vi "DSF.Engine.Transfer.Create.vi"(5 "id":i32, 7 "channel blocks":T1[](array[typedef]) {"buffer offset" format="%d bytes"}, 8 "error in (no error)":errorcluster, 9 "String Buffer":refnum<class "DSF.Engine.Memory.Buffer.lvclass">, 10 "Intermediate Buffer":refnum<class "DSF.Engine.Pointer.DBL.lvclass">, 11 "Inline Buffer":refnum<class "DSF.Engine.Pointer.DBL.lvclass">) -> (0 "error out":errorcluster, 3 "Transfer out":refnum<class "DSF.Engine.Transfer.lvclass">)   [LabVIEW 2017, in "DSF.Engine.lvlib" / "DSF.Engine.Transfer.lvclass"]
uses:
  DSF.Engine.Transfer.lvclass
  Buffer/DSF.Engine.Memory.Buffer.lvclass
  Pointer/DSF.Engine.Pointer.DBL.lvclass
  Shared/Typedefs/DSF Runtime Channel Block.ctl
  DSF Configuration API/1.0.0/Public/Controls/DSF Data Type.ctl
  DSF.Engine.Transfer.lvclass/DSF.Engine.Transfer.ctl
  DSF.Engine.lvlib
  DSF Configuration API/1.0.0/DSF Configuration API.lvlib
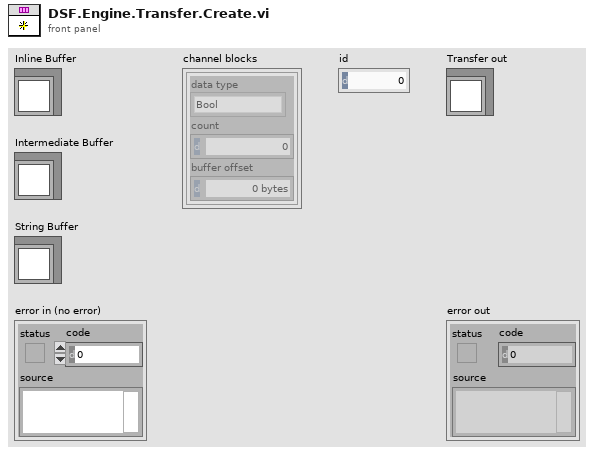
[diagram p1: front panel]
types:
  T1 = typedef "DSF.Engine.lvlib/DSF Runtime Channel Block.ctl" = cluster{"data type":T2, "count":u64, "buffer offset":u64}
  T2 = typedef "DSF Configuration API.lvlib/DSF Data Type.ctl" = enum8{"Bool", "SGL", "DBL", "I8", "I16", "I32", "I64", "U8", "U16", "U32", "U64"}
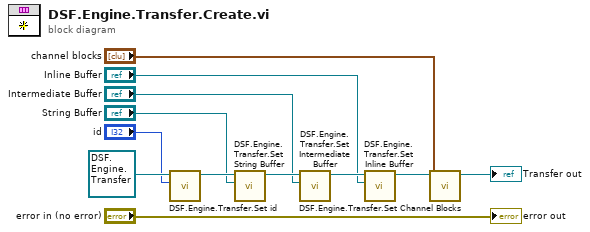
[diagram p0: block diagram]
diagram:
  n1 = call "DSF.Engine.Transfer.Set id.vi"("id"="id", "Transfer in"=refnum<class "DSF.Engine.Transfer.lvclass"> refnum) -> ("Transfer out"=w12:refnum<class "DSF.Engine.Transfer.lvclass">)  [unwired: 9 in]
  n2 = call "DSF.Engine.Transfer.Set String Buffer.vi"("Buffer"="String Buffer", "Transfer in"=w12) -> ("Transfer out"=w11:refnum<class "DSF.Engine.Transfer.lvclass">)  [unwired: 9 in]
  n3 = call "DSF.Engine.Transfer.Set Intermediate Buffer.vi"("DBL Buffer"="Intermediate Buffer", "Transfer in"=w11) -> ("Transfer out"=w10:refnum<class "DSF.Engine.Transfer.lvclass">)  [unwired: 9 in]
  n4 = call "DSF.Engine.Transfer.Set Inline Buffer.vi"("Inline Buffer"="Inline Buffer", "Transfer in"=w10) -> ("Transfer out"=w3:refnum<class "DSF.Engine.Transfer.lvclass">)  [unwired: 9 in]
  n5 = call "DSF.Engine.Transfer.Set Channel Blocks.vi"("channel blocks"="channel blocks", "Transfer in"=w3) -> ("Transfer out"=→"Transfer out":refnum<class "DSF.Engine.Transfer.lvclass">)  [unwired: 9 in]
  "error out" <- "error in (no error)"
